vi "Insert Into Array (Single String).vi"(9 "index":i32, 10 "String":string, 11 "JSON Array in":refnum<class "JSON Helper.lvclass">) -> (3 "JSON Array out":refnum<class "JSON Helper.lvclass">)   [LabVIEW 2016, in "JSON Helper.lvclass"]
doc: "Inserts an element or subarray into a JSON array at the point you specify in index."
uses:
  JSON Helper/JSON Helper.lvclass
  JSON String/New JSON String.vi
  Insert Into Array (Single).vi
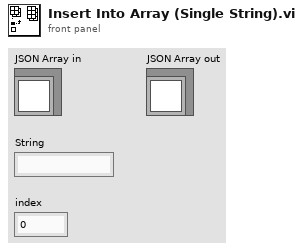
[diagram p1: front panel]
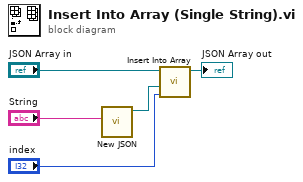
[diagram p0: block diagram]
diagram:
  n1 = call-poly "New JSON.vi"("value"="String") -> ("JSON String out"=w2:refnum<class "JSON Helper.lvclass">)  [unwired: 9 in, 1 out]
  n2 = call-poly "Insert Into Array.vi"("index"="index", "JSON Object in"=w2, "JSON Array in"="JSON Array in") -> ("JSON Array out"=→"JSON Array out":refnum<class "JSON Helper.lvclass">)  [unwired: 8 in]
